vi "VIEW.vi"() -> ()   [LabVIEW 2013]
uses:
  base/VIEW.lvclass
  Controller/base/CONTROLLER.lvclass
panel:
  in  "ctrl2":string
  in  "DoAction1":bool
  in  "mystring":string
  in  "Enqueue Element":bool
  in  "stop":bool
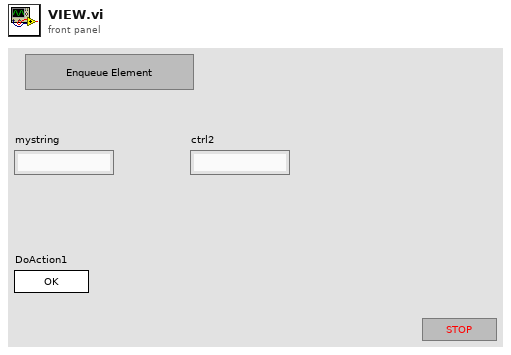
[diagram p1: front panel]
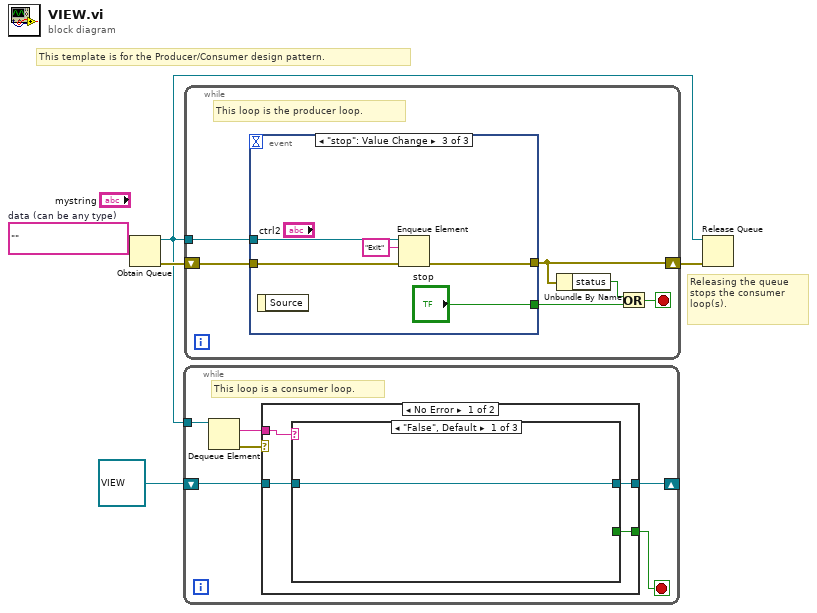
[diagram p0: block diagram]
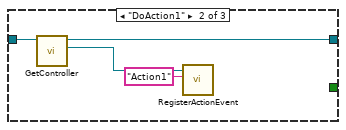
[diagram p2: hidden frame]
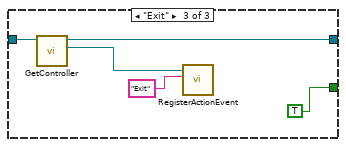
[diagram p3: hidden frame]
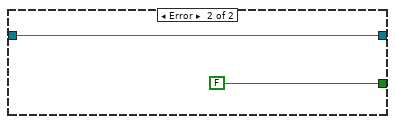
[diagram p4: hidden frame]
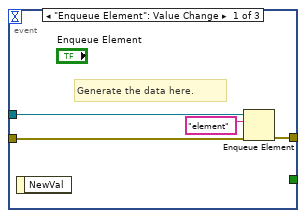
[diagram p5: hidden frame]
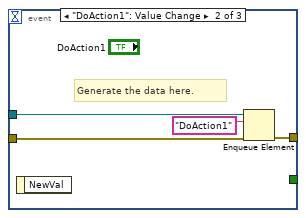
[diagram p6: hidden frame]
diagram:
  w3 = ""  # data (can be any type)
  # "Releasing the queue stops the consumer loop(s)."
  # "This template is for the Producer/Consumer design pattern."
  n1 = Obtain Queue(element data type=w3) -> (queue out=w2:refnum<queue>, error out=w5:errorcluster)  [unwired: 4 in, 1 out]
  n2 = while {
    tunnel: w2 -> [w11]
    shift-right: [w6] -> _
    shift-left: refnum<class "VIEW.lvclass"> refnum ("VIEW.lvclass") -> [w7]
    stop <- w8 stop-if-true
    # "This loop is a consumer loop."
    n3 = Dequeue Element(queue=w11) -> (element=w9:string, error out=w10:errorcluster)  [unwired: 2 in, 2 out]
    n4 = case shown="No Error" w10 {
      tunnel: w9 -> [w15 _]
      tunnel: [w12 FALSE] -> w8
      tunnel: w7 -> [w14 w26]
      tunnel: [w13 w26] -> w6
      frame No Error {
        n5 = case shown="\"False\", Default" w15 {
          tunnel: w14 -> [w16 w20 w25]
          tunnel: [w16 w18 w23] -> w13
          tunnel: [_ _ TRUE] -> w12
          frame "False", Default {
          }
          frame "DoAction1" {
            n6 = call-dynamic "GetController.vi"("VIEW in"=w20) -> ("CONTROLLER"=w19:refnum<class "CONTROLLER.lvclass">, "VIEW out"=w18:refnum<class "VIEW.lvclass">)  [unwired: 8 in, 1 out]
            n7 = call "RegisterActionEvent.vi"("Action"="Action1", "CONTROLLER in"=w19) -> ()  [unwired: 8 in, 2 out]
          }
          frame "Exit" {
            n8 = call-dynamic "GetController.vi"("VIEW in"=w25) -> ("CONTROLLER"=w24:refnum<class "CONTROLLER.lvclass">, "VIEW out"=w23:refnum<class "VIEW.lvclass">)  [unwired: 8 in, 1 out]
            n9 = call "RegisterActionEvent.vi"("Action"="Exit", "CONTROLLER in"=w24) -> ()  [unwired: 8 in, 2 out]
          }
        }
      }
      frame Error {
      }
    }
  }
  n10 = while {
    shift-right: [w29] -> w4
    shift-left: w5 -> [w32]
    tunnel: w2 -> [w33]
    stop <- w30 stop-if-true
    # "This loop is the producer loop."
    n11 = event shown="[2] \"stop\": Value Change" {
      selector: _ -> [_ _ _]
      dyn-events: _ -> [_ _ _]
      timeout: _ -> [_ _ _]
      tunnel: w33 -> [w37 w41 w43]
      tunnel: w32 -> [w36 w40 w45]
      tunnel: [w35 w39 w44] -> w29
      tunnel: [_ _ "stop"] -> w31
      event "Enqueue Element": Value Change {
        # "Generate the data here."
        n12 = event-data() -> ()  [unwired: 1 in, 1 out]
        n13 = Enqueue Element(queue=w37, element="element", error in (no error)=w36) -> (error out=w35:errorcluster)  [unwired: 1 in, 2 out]
      }
      event "DoAction1": Value Change {
        # "Generate the data here."
        n14 = event-data() -> ()  [unwired: 1 in, 1 out]
        n15 = Enqueue Element(queue=w41, element="DoAction1", error in (no error)=w40) -> (error out=w39:errorcluster)  [unwired: 1 in, 2 out]
      }
      event "stop": Value Change {
        n16 = event-data() -> ()  [unwired: 1 in, 1 out]
        n17 = Enqueue Element(queue=w43, element="Exit", error in (no error)=w45) -> (error out=w44:errorcluster)  [unwired: 1 in, 2 out]
      }
    }
    n18 = Unbundle By Name(w29) -> ("status"=w28:bool)
    n19 = Or(x=w28, y=w31) -> (x .or. y?=w30:bool)
  }
  n20 = Release Queue(queue=w2, error in (no error)=w4) -> ()  [unwired: 1 in, 3 out]
